vi "发射.vi"() -> ()   [LabVIEW 2018]
uses:
  <vilib>/Instr/_visa.llb/VISA Configure Serial Port (Instr).vi
  <vilib>/measure/NI_MABase.lvlib
panel:
  in  "波特率":u16
  in  "VISA资源":refnum<visa-resource-name>
  out "通讯结束":bool[](array[boolean])
  out "字节3":bool[](array[boolean])
  out "通讯中":bool[](array[boolean])
  out "字节2":bool[](array[boolean])
  out "字节1":bool[](array[boolean])
  in  "波形频率":u16(ring) items=["16"=1, "32"=2, "48"=3, "64"=4, "80"=5, "96"=6, "112"=7, "128"=8, "144"=9, "160"=10, "176"=11, "192"=12, "208"=13, "224"=14, "240"=15, "256"=16, "272"=17, "288"=18, "304"=19, "320"=20, "336"=21, "352"=22, "368"=23, "384"=24, "400"=25, "416"=26, "432"=27, "448"=28, "464"=29, "496"=31, "512"=32, "544"=34, "624"=39, "656"=41, "704"=44, "768"=48, "832"=52, "896"=56, "992"=62]
  in  "校对码":u8
  in  "波形类型":enum16{"互补", "非互补"}(ring)
  out "发送的波形":waveform(dbl)[](graph)
  in  "发射":bool
  in  "停止":bool caption="STOP"
  # "地学虚拟仪器发射模块"
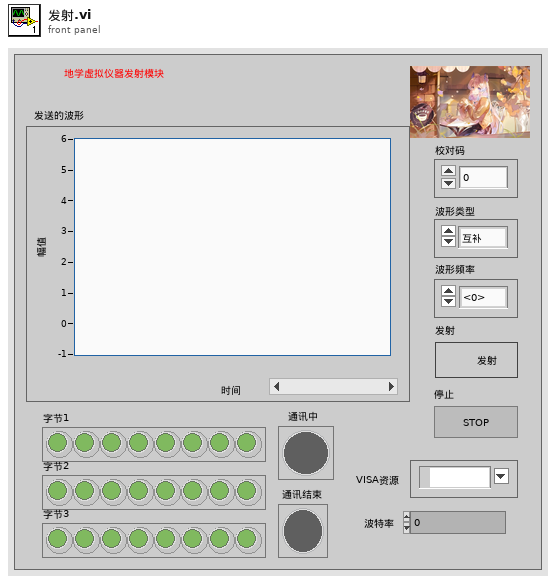
[diagram p1: front panel]
types:
  T1 = enum16{"None", "Odd", "Even", "Mark", "Space", "COM1"}
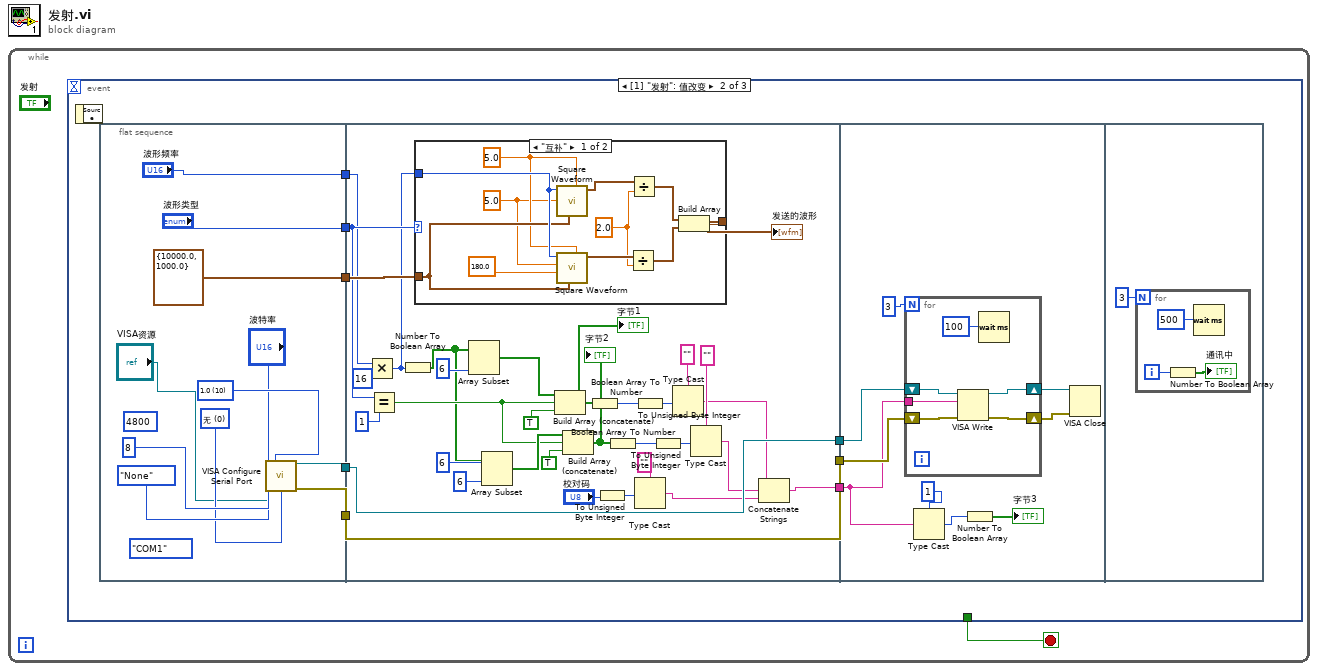
[diagram p0: block diagram]
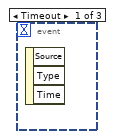
[diagram p2: hidden frame]
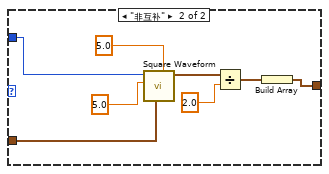
[diagram p3: hidden frame]
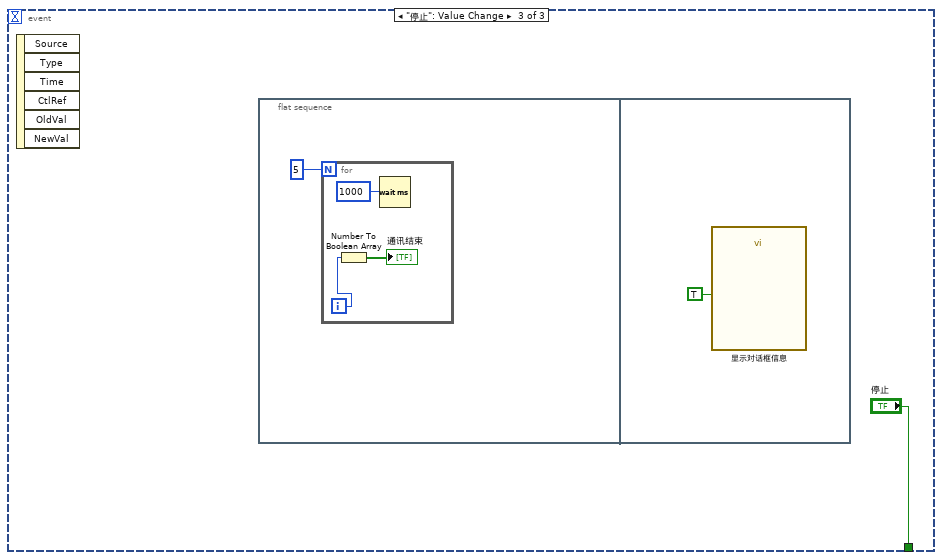
[diagram p4: hidden frame]
diagram:
  n1 = while {
    stop <- w1 stop-if-true
    n2 = event shown="[1] \"发射\": 值改变" {
      selector: _ -> [_ _ _]
      dyn-events: _ -> [_ _ _]
      timeout: _ -> [_ _ _]
      tunnel: [_ _ "停止"] -> w1
      event Timeout {
        n3 = event-data() -> ()  [unwired: 1 in, 3 out]
      }
      event "发射": Value Change {
        n4 = event-data() -> ()  [unwired: 1 in, 1 out]
        n5 = flat-sequence {
          tunnel: ["波形频率"] -> w9
          tunnel: ["波形类型"] -> w8
          tunnel: [cluster{dbl, dbl} {10000.0, 1000.0}] -> w7
          tunnel: [w17] -> w6
          tunnel: [w16] -> w5
          tunnel: w9 -> [w29]
          tunnel: w8 -> [w52]
          tunnel: w7 -> [w53]
          tunnel: w6 -> [w43]
          tunnel: w5 -> [w42]
          tunnel: [w43] -> w4
          tunnel: [w42] -> w3
          tunnel: [w32] -> w2
          tunnel: w4 -> [w80]
          tunnel: w3 -> [w79]
          tunnel: w2 -> [w74]
          frame #0 {
            (unwired) enum16{"COM1"}."COM1"
            w15 = u16 0 items=["无", "XON/XOFF", "RTS/CTS", "XON/XOFF & RTS/CTS", "DTR/DSR", "XON/XOFF & DTR/DSR"] ("flow control (0:none)")
            w18 = u16 10 items=["1.0"=10, "1.5"=15, "2.0"=20] ("stop bits (10: 1 bit)")
            (unwired) u32 4800 ("baud rate (9600)")
            n6 = call-poly "VISA Configure Serial Port"("VISA resource name"="VISA资源", "baud rate (9600)"="波特率", "data bits (8)"=u16 8, "parity (0:none)"=T1."None", "stop bits (10: 1 bit)"=w18, "flow control (0:none)"=w15) -> ("VISA resource name out"=w17:refnum<visa-resource-name>, "error out"=w16:errorcluster)  [unwired: 8 in]
          }
          frame #1 {
            n7 = Multiply(x=w29, y=u32 16) -> (x*y=w25:u32)
            n8 = Equal?(x=w52, y=u16 1) -> (x = y?=w22:bool)
            n9 = Number To Boolean Array(number=w25) -> (Boolean array=w21:bool[])
            n10 = case shown="\"互补\"" w52 {
              tunnel: w53 -> [w63 w69]
              tunnel: w25 -> [w64 w72]
              tunnel: [w54 w65] -> w24
              frame "互补" {
                w57 = 2.0
                w61 = 5.0
                w62 = 5.0
                n11 = call <vilib>:"Square Waveform.vi"("offset"=w62, "sampling info"=w63, "amplitude"=w61, "frequency"=w64) -> ("signal out"=w59:waveform(dbl))  [unwired: 6 in, 1 out]
                n12 = call <vilib>:"Square Waveform.vi"("offset"=w62, "sampling info"=w63, "phase"=180.0, "amplitude"=w61, "frequency"=w64) -> ("signal out"=w58:waveform(dbl))  [unwired: 5 in, 1 out]
                n13 = Divide(x=w58, y=w57) -> (x/y=w55:waveform(dbl))
                n14 = Divide(x=w59, y=w57) -> (x/y=w56:waveform(dbl))
                n15 = Build Array(w56, w55) -> (w54:waveform(dbl)[])
              }
              frame "非互补" {
                n16 = call <vilib>:"Square Waveform.vi"("offset"=5.0, "sampling info"=w69, "amplitude"=5.0, "frequency"=w72) -> ("signal out"=w68:waveform(dbl))  [unwired: 6 in, 1 out]
                n17 = Divide(x=w68, y=2.0) -> (x/y=w66:waveform(dbl))
                n18 = Build Array(w66) -> (w65:waveform(dbl)[])
              }
            }
            "发送的波形" <- w24
            n19 = Array Subset(array=w21, length=6 ("长度")) -> (w49:bool[])  [unwired: 1 in]
            n20 = Array Subset(array=w21, index=6 ("索引"), length=6 ("长度")) -> (w36:bool[])
            n21 = Build Array (concatenate)(w49, w22, TRUE ("元素")) -> (w47:bool[])
            "字节1" <- w47
            n22 = Build Array (concatenate)(w36, w22, TRUE ("元素")) -> (w39:bool[])
            "字节2" <- w39
            n23 = Boolean Array To Number(Boolean array=w47) -> (number=w46:u32)
            n24 = To Unsigned Byte Integer(number="校对码") -> (unsigned 8bit integer=w27:u8)
            n25 = Boolean Array To Number(Boolean array=w39) -> (number=w38:u32)
            n26 = To Unsigned Byte Integer(number=w46) -> (unsigned 8bit integer=w45:u8)
            n27 = Type Cast(type="" ("类型"), x=w27) -> (*(type *) &x=w26:string)
            n28 = To Unsigned Byte Integer(number=w38) -> (unsigned 8bit integer=w37:u8)
            n29 = Type Cast(type="" ("类型"), x=w45) -> (*(type *) &x=w34:string)
            n30 = Type Cast(type="" ("类型"), x=w37) -> (*(type *) &x=w28:string)
            n31 = Concatenate Strings(w34, w28, w26) -> (w32:string)
          }
          frame #2 {
            n32 = for {
              N: 3 -> [_]
              tunnel: w74 -> [w87]
              shift-right: [w84] -> w77
              shift-left: w80 -> [w86]
              shift-right: [w83] -> w78
              shift-left: w79 -> [w85]
              n33 = VISA Write(VISA resource name=w86, write buffer=w87, error in (no error)=w85) -> (VISA resource name out=w84:refnum<visa-resource-name>, error out=w83:errorcluster)  [unwired: 1 out]
              n34 = Wait (ms)(milliseconds to wait=u32 100 ("等待时间（毫秒）")) -> ()  [unwired: 1 out]
            }
            n35 = Type Cast(type=1, x=w74) -> (*(type *) &x=w76:i32)
            n36 = Number To Boolean Array(number=w76) -> (Boolean array=→"字节3":bool[])
            n37 = VISA Close(VISA resource name=w77, error in (no error)=w78) -> ()  [unwired: 1 out]
          }
          frame #3 {
            n38 = for {
              N: 3 -> [_]
              i -> [w90]
              n39 = Number To Boolean Array(number=w90) -> (Boolean array=→"通讯中":bool[])
              n40 = Wait (ms)(milliseconds to wait=u32 500 ("等待时间（毫秒）")) -> ()  [unwired: 1 out]
            }
          }
        }
      }
      event "停止": Value Change {
        n41 = event-data() -> ()  [unwired: 1 in, 6 out]
        n42 = flat-sequence {
          frame #0 {
            n43 = for {
              N: 5 -> [_]
              i -> [w95]
              n44 = Number To Boolean Array(number=w95) -> (Boolean array=→"通讯结束":bool[])
              n45 = Wait (ms)(milliseconds to wait=u32 1000 ("等待时间（毫秒）")) -> ()  [unwired: 1 out]
            }
          }
          frame #1 {
            n46 = call "显示对话框信息"("Enable"=TRUE) -> ()  [unwired: 9 in, 2 out]
          }
        }
      }
    }
  }
